vi "DAQ Initialize.vi"(8 "error in":errorcluster) -> (0 "error out":errorcluster, 3 "DAQmx Task Name":refnum<k21>)   [LabVIEW 2019]
uses:
  <vilib>/DAQmx/create/channels.llb/DAQmx Create Channel (AI-Voltage-Basic).vi
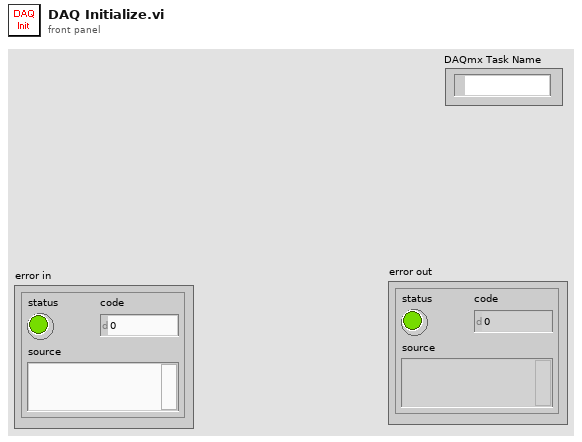
[diagram p1: front panel]
types:
  T1 = typedef "Device Settings.ctl" = cluster{"Device Type":string, "Device Name":string, "DAQmx Name":tag, "Terminal Wiring":i32}
  T2 = cluster{"TagId":string, "TagName":string, "TagType":string, "PhysicalChannel":tag, "Vmin":dbl, "Vmax":dbl, "Unit":string, "EUmin":dbl, "EUmax":dbl}[]
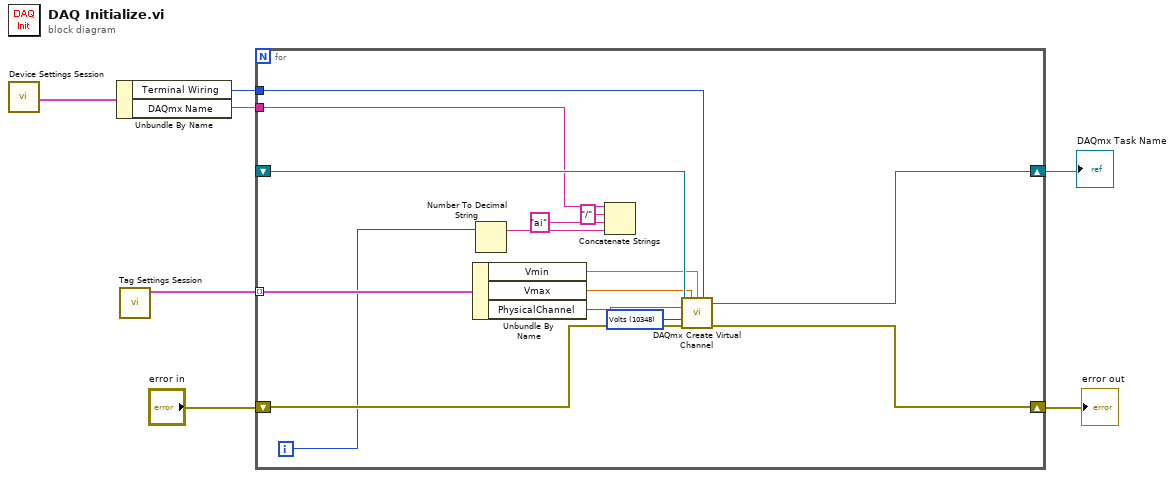
[diagram p0: block diagram]
diagram:
  n1 = call "Device Settings Session.vi"() -> ("Device Settings"=w3:T1)  [unwired: 2 in, 1 out]
  n2 = Unbundle By Name(w3) -> ("Terminal Wiring"=w2:i32, "DAQmx Name"=w1:tag)
  n3 = call "Tag Settings Session.vi"() -> ("Tag Settings"=w4:T2)  [unwired: 10 in, 1 out]
  n4 = for {
    tunnel: w4 -> [w22] mode=indexing
    shift-right: [w21] -> w5
    shift-left: _ -> [w20]
    shift-right: [w18] -> w6
    shift-left: "error in" -> [w19]
    tunnel: w2 -> [w9]
    tunnel: w1 -> [w8]
    i -> [w17]
    w13 = 10348 items=["Volts"=10348, "From Custom Scale"=10065] ("units")
    n5 = Unbundle By Name(w22) -> ("Vmin"=w16:dbl, "Vmax"=w15:dbl, "PhysicalChannel"=w10:tag)
    n6 = Number To Decimal String(number=w17) -> (decimal integer string=w11:string)  [unwired: 1 in]
    n7 = Concatenate Strings(w8, "/" ("string"), "ai" ("Physical Channel"), w11) -> ()  [unwired: 1 out]
    n8 = call-poly <vilib>:"DAQmx Create Virtual Channel.vi"("task in"=w20, "maximum value"=w15, "minimum value"=w16, "input terminal configuration"=w9, "physical channels"=w10, "units"=w13, "error in"=w19) -> ("task out"=w21:refnum<k21>, "error out"=w18:errorcluster)  [unwired: 7 in]
  }
  "error out" <- w6
  "DAQmx Task Name" <- w5
